vi "Get Initial Values.vi"(8 "error in (no error)":errorcluster, 11 "VISA resource name":refnum<visa-resource-name>) -> (0 "error out":errorcluster, 2 "initial values":T1={"frequency"=0.0, "average"=0, "voltage"=0.0, "units"=1, "dev mode"=FALSE, "dev point auto"={"dev point auto cap"=FALSE, "dev point auto loss"=FALSE}, "dev parameters"={"dev bounds"={"dev bound upper cap"=0.0, "dev bound upper loss"=0.0, "dev bound lower cap"=0.0, "dev bound lower loss"=0.0}, "dev point"={"dev point cap"=0.0, "dev point loss"=0.0}, "dev position"={"dev position cap"=0.0, "dev position loss"=0.0}, "dev span"={"dev span cap"=0.0, "dev span loss"=0.0}, "dev margin"=0.0}, "dev average"=0.0, "dev format"={"dev format cap"=0, "dev format loss"=0}, "dev rollofff"={"dev rolloff setting"=0.0, "dev rolloff actual"=0.0}, "aout bias"={"ABiasC"=0.0, "ABiasL"=0.0}, "aout bounds"={"ABndUpC"=0.0, "ABndUpL"=0.0, "ABndLoC"=0.0, "ABndLoL"=0.0}, "aout cfactor"={"CFactorC"=0.0, "CFactorL"=0.0}, "aout limit error"={"ALimErrC"=FALSE, "ALimErrL"=FALSE}, "aout limit"={"ALimUpC"=0.0, "ALimUpL"=0.0, "ALimLoC"=0.0, "ALimLoL"=0.0}, "aout source"={"ASourceC (0:DEV)"=0, "ASourceL (0:DEV)"=0}, "aout span"={"ASpanC (20.0)"=20.0, "ASpanL (20.0)"=20.0}, "aout point"={"APointC"=20.0, "APointL"=20.0}} {"aout source"."ASourceL (0:DEV)" items=["DEV", "BIAS", "GROUND"]; "aout source"."ASourceC (0:DEV)" items=["DEV", "BIAS", "GROUND"]; "units" items=["NS"=1, "DS"=2, "KO"=3, "GO"=4, "JP"=5]}, 3 "VISA resource name out":refnum<visa-resource-name>)   [LabVIEW 2019, in "Andeen-Hagerling 2700A.lvlib"]
uses:
  Andeen-Hagerling 2700A.lvlib
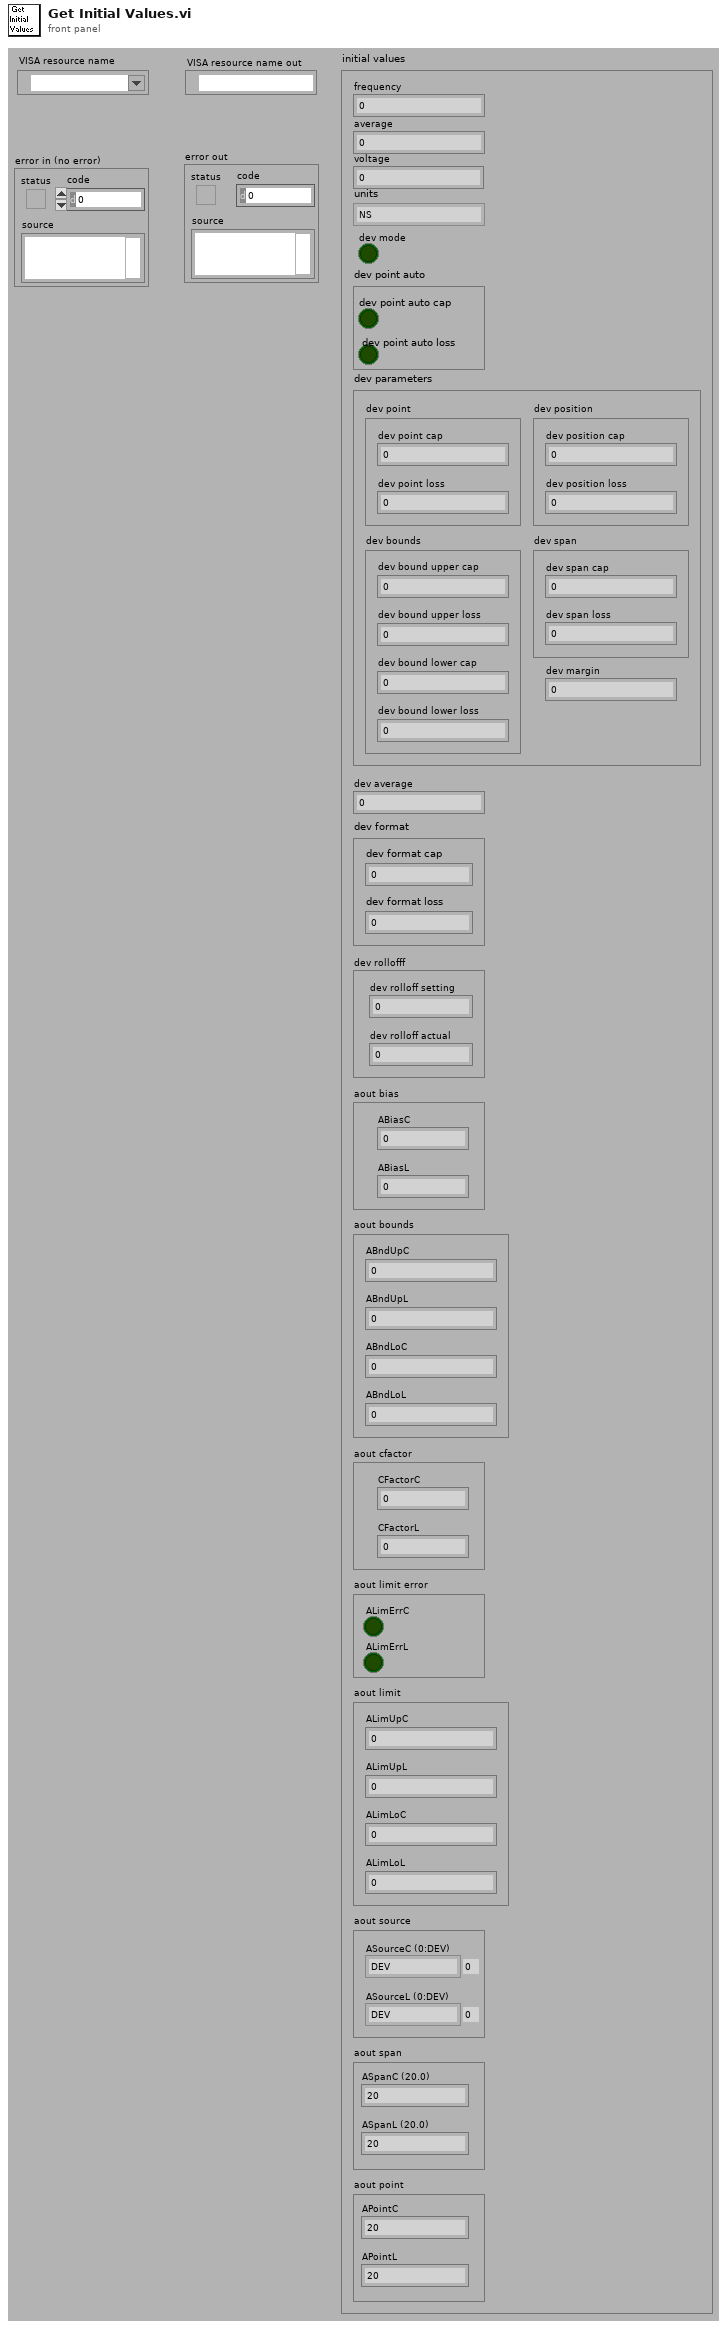
[diagram p1: front panel]
types:
  T1 = cluster{"frequency":dbl, "average":i32, "voltage":dbl, "units":i32, "dev mode":bool, "dev point auto":cluster{"dev point auto cap":bool, "dev point auto loss":bool}, "dev parameters":cluster{"dev bounds":cluster{"dev bound upper cap":dbl, "dev bound upper loss":dbl, "dev bound lower cap":dbl, "dev bound lower loss":dbl}, "dev point":cluster{"dev point cap":dbl, "dev point loss":dbl}, "dev position":cluster{"dev position cap":dbl, "dev position loss":dbl}, "dev span":cluster{"dev span cap":dbl, "dev span loss":dbl}, "dev margin":dbl}, "dev average":dbl, "dev format":cluster{"dev format cap":i32, "dev format loss":i32}, "dev rollofff":cluster{"dev rolloff setting":dbl, "dev rolloff actual":dbl}, "aout bias":cluster{"ABiasC":dbl, "ABiasL":dbl}, "aout bounds":cluster{"ABndUpC":dbl, "ABndUpL":dbl, "ABndLoC":dbl, "ABndLoL":dbl}, "aout cfactor":cluster{"CFactorC":dbl, "CFactorL":dbl}, "aout limit error":cluster{"ALimErrC":bool, "ALimErrL":bool}, "aout limit":cluster{"ALimUpC":dbl, "ALimUpL":dbl, "ALimLoC":dbl, "ALimLoL":dbl}, "aout source":cluster{"ASourceC (0:DEV)":u16, "ASourceL (0:DEV)":u16}, "aout span":cluster{"ASpanC (20.0)":dbl, "ASpanL (20.0)":dbl}, "aout point":cluster{"APointC":dbl, "APointL":dbl}}
  T2 = cluster{"dev point auto cap":bool, "dev point auto loss":bool}
  T3 = cluster{"dev bounds":cluster{"dev bound upper cap":dbl, "dev bound upper loss":dbl, "dev bound lower cap":dbl, "dev bound lower loss":dbl}, "dev point":cluster{"dev point cap":dbl, "dev point loss":dbl}, "dev position":cluster{"dev position cap":dbl, "dev position loss":dbl}, "dev span":cluster{"dev span cap":dbl, "dev span loss":dbl}, "dev margin":dbl}
  T4 = cluster{"dev format cap":i32, "dev format loss":i32}
  T5 = cluster{"dev rolloff setting":dbl, "dev rolloff actual":dbl}
  T6 = cluster{"ABndUpC":dbl, "ABndUpL":dbl, "ABndLoC":dbl, "ABndLoL":dbl}
  T7 = cluster{"ALimUpC":dbl, "ALimUpL":dbl, "ALimLoC":dbl, "ALimLoL":dbl}
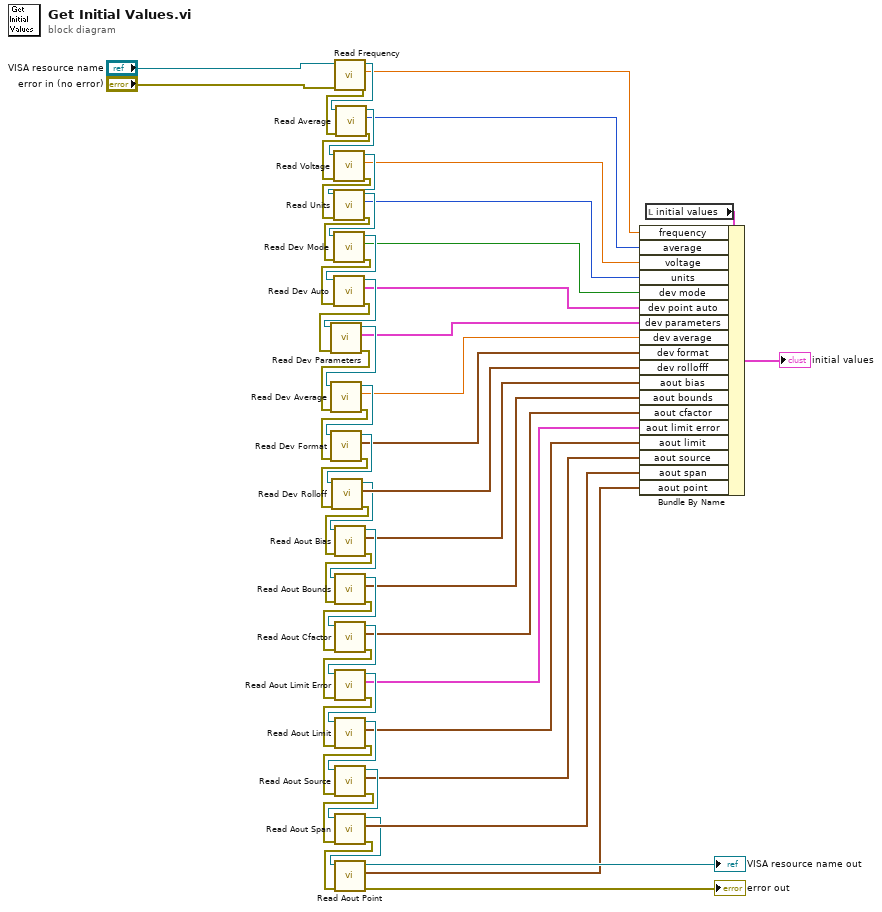
[diagram p0: block diagram]
diagram:
  n1 = call "Read Frequency.vi"("error in (no error)"="error in (no error)", "VISA resource name"="VISA resource name") -> ("error out"=w55:errorcluster, "frequency"=w37:dbl, "VISA resource name out"=w56:refnum<visa-resource-name>)  [unwired: 7 in]
  n2 = call "Read Average.vi"("error in (no error)"=w55, "VISA resource name"=w56) -> ("error out"=w57:errorcluster, "average"=w36:i32, "VISA resource name out"=w58:refnum<visa-resource-name>)  [unwired: 7 in]
  n3 = call "Read Voltage.vi"("error in (no error)"=w57, "VISA resource name"=w58) -> ("error out"=w53:errorcluster, "voltage"=w35:dbl, "VISA resource name out"=w54:refnum<visa-resource-name>)  [unwired: 7 in]
  n4 = call "Read Units.vi"("error in (no error)"=w53, "VISA resource name"=w54) -> ("error out"=w51:errorcluster, "units"=w34:i32, "VISA resource name out"=w52:refnum<visa-resource-name>)  [unwired: 7 in]
  n5 = call "Read Dev Mode.vi"("error in (no error)"=w51, "VISA resource name"=w52) -> ("error out"=w50:errorcluster, "dev mode"=w33:bool, "VISA resource name out"=w49:refnum<visa-resource-name>)  [unwired: 7 in]
  n6 = call "Read Dev Auto.vi"("error in (no error)"=w50, "VISA resource name"=w49) -> ("error out"=w48:errorcluster, "dev point auto"=w32:T2, "VISA resource name out"=w47:refnum<visa-resource-name>)  [unwired: 7 in]
  n7 = call "Read Dev Parameters.vi"("error in (no error)"=w48, "VISA resource name"=w47) -> ("error out"=w45:errorcluster, "dev parameters"=w31:T3, "VISA resource name out"=w46:refnum<visa-resource-name>)  [unwired: 7 in]
  n8 = call "Read Dev Average.vi"("error in (no error)"=w45, "VISA resource name"=w46) -> ("error out"=w44:errorcluster, "dev average"=w30:dbl, "VISA resource name out"=w43:refnum<visa-resource-name>)  [unwired: 7 in]
  n9 = call "Read Dev Format.vi"("error in (no error)"=w44, "VISA resource name"=w43) -> ("error out"=w41:errorcluster, "dev format"=w29:T4, "VISA resource name out"=w42:refnum<visa-resource-name>)  [unwired: 7 in]
  n10 = call "Read Dev Rolloff.vi"("error in (no error)"=w41, "VISA resource name"=w42) -> ("error out"=w13:errorcluster, "dev rollofff"=w28:T5, "VISA resource name out"=w26:refnum<visa-resource-name>)  [unwired: 7 in]
  n11 = call "Read Aout Bias.vi"("error in (no error)"=w13, "VISA resource name"=w26) -> ("error out"=w24:errorcluster, "aout bias"=w12:cluster{"ABiasC":dbl, "ABiasL":dbl}, "VISA resource name out"=w25:refnum<visa-resource-name>)  [unwired: 7 in]
  n12 = call "Read Aout Bounds.vi"("error in (no error)"=w24, "VISA resource name"=w25) -> ("error out"=w22:errorcluster, "aout bounds"=w11:T6, "VISA resource name out"=w23:refnum<visa-resource-name>)  [unwired: 7 in]
  n13 = call "Read Aout Cfactor.vi"("error in (no error)"=w22, "VISA resource name"=w23) -> ("error out"=w20:errorcluster, "aout cfactor"=w10:cluster{"CFactorC":dbl, "CFactorL":dbl}, "VISA resource name out"=w21:refnum<visa-resource-name>)  [unwired: 7 in]
  n14 = call "Read Aout Limit Error.vi"("error in (no error)"=w20, "VISA resource name"=w21) -> ("error out"=w18:errorcluster, "aout limit error"=w9:cluster{"ALimErrC":bool, "ALimErrL":bool}, "VISA resource name out"=w19:refnum<visa-resource-name>)  [unwired: 7 in]
  n15 = call "Read Aout Limit.vi"("error in (no error)"=w18, "VISA resource name"=w19) -> ("error out"=w16:errorcluster, "aout limit"=w8:T7, "VISA resource name out"=w17:refnum<visa-resource-name>)  [unwired: 7 in]
  n16 = call "Read Aout Source.vi"("error in (no error)"=w16, "VISA resource name"=w17) -> ("error out"=w14:errorcluster, "aout source"=w7:cluster{"ASourceC":u16, "ASourceL":u16}, "VISA resource name out"=w15:refnum<visa-resource-name>)  [unwired: 7 in]
  n17 = call "Read Aout Span.vi"("error in (no error)"=w14, "VISA resource name"=w15) -> ("error out"=w4:errorcluster, "aout span"=w6:cluster{"ASpanC":dbl, "ASpanL":dbl}, "VISA resource name out"=w5:refnum<visa-resource-name>)  [unwired: 7 in]
  n18 = call "Read Aout Point.vi"("error in (no error)"=w4, "VISA resource name"=w5) -> ("error out"=→"error out":errorcluster, "aout point"=w1:cluster{"APointC":dbl, "APointL":dbl}, "VISA resource name out"=→"VISA resource name out":refnum<visa-resource-name>)  [unwired: 7 in]
  n19 = local read "initial values"() -> (w38:T1)
  n20 = Bundle By Name(cluster=w38, "frequency"=w37, "average"=w36, "voltage"=w35, "units"=w34, "dev mode"=w33, "dev point auto"=w32, "dev parameters"=w31, "dev average"=w30, "dev format"=w29, "dev rollofff"=w28, "aout bias"=w12, "aout bounds"=w11, "aout cfactor"=w10, "aout limit error"=w9, "aout limit"=w8, "aout source"=w7, "aout span"=w6, "aout point"=w1) -> (→"initial values":T1)
